vi "MAT Search Matrix.vi"(7 "offset in (-1: current position)":i64=-1, 8 "Error In":errorcluster, 10 "matrix name":string, 11 "Ref Num":refnum<file>) -> (0 "error out":errorcluster, 3 "Dup Ref Num":refnum<file>)   [LabVIEW 2013]
doc: "Searches matrix offset in the MAT file. It will set the read pointer to start of the matrix header."
uses:
  <vilib>/Utility/error.llb/Error Cluster From Error Code.vi
  <vilib>/ErrorRing/Error Ring.xnode
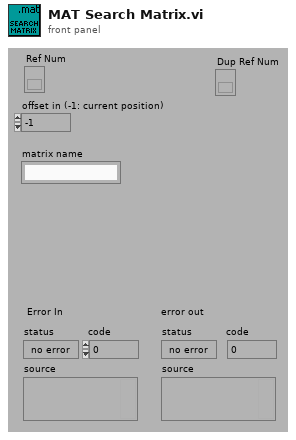
[diagram p1: front panel]
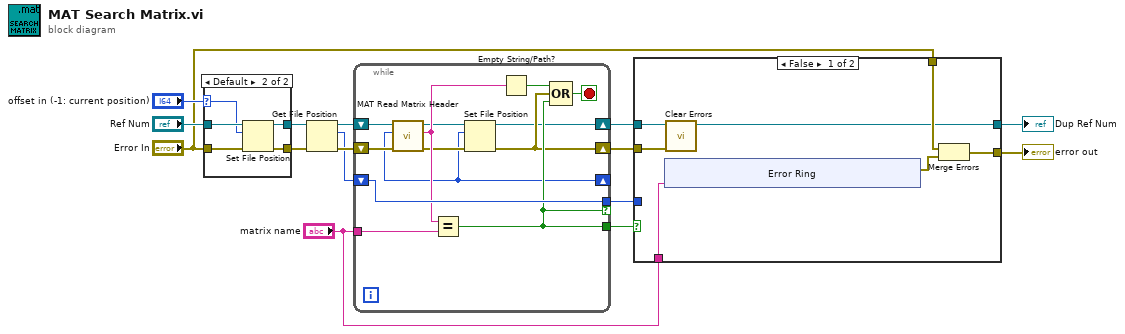
[diagram p0: block diagram]
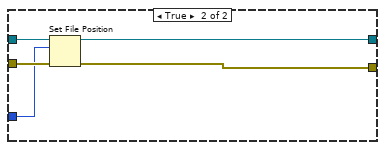
[diagram p2: hidden frame]
diagram:
  n1 = case shown="Default" "offset in (-1: current position)" {
    selector: "offset in (-1: current position)" -> [_ w18]
    tunnel: "Error In" -> [w16 w22]
    tunnel: [w16 w21] -> w13
    tunnel: [w17 w20] -> w12
    tunnel: "Ref Num" -> [w17 w19]
    frame -1 {
    }
    frame Default {
      n2 = Set File Position(offset (in bytes) (0)=w18, refnum=w19, error in=w22) -> (refnum out=w20:refnum<file>, error out=w21:errorcluster)  [unwired: 1 in]
    }
  }
  n3 = Get File Position(4:w13, 7:w12) -> (0:w11:errorcluster, 2:w9:i64, 3:w10:refnum<file>)
  n4 = while {
    shift-right: [w26] -> w7
    shift-left: w11 -> [w35]
    shift-right: [w24] -> w6
    shift-left: w10 -> [w34]
    shift-right: [w23] -> _
    shift-left: w9 -> [w32]
    tunnel: "matrix name" -> [w33]
    tunnel: [w32] -> w5 if=w28
    tunnel: [w28] -> w8
    stop <- w29 stop-if-true
    n5 = call "MAT Read Matrix Header.vi"("Error In"=w35, "Ref Num"=w34) -> ("error out"=w27:errorcluster, "Matrix Name"=w30:string, "Dup Ref Num"=w25:refnum<file>, "next variable offset"=w23:i64)  [unwired: 1 in, 5 out]
    n6 = Equal?(x=w30, y=w33) -> (x = y?=w28:bool)
    n7 = Set File Position(offset (in bytes) (0)=w23, refnum=w25, error in=w27) -> (refnum out=w24:refnum<file>, error out=w26:errorcluster)  [unwired: 1 in]
    n8 = Empty String/Path?(string/path=w30) -> (empty?=w31:bool)
    n9 = Compound Arithmetic op=OR(w31, w26, w28) -> (w29:bool)
  }
  n10 = case shown="False" w8 {
    tunnel: w7 -> [w37 w53]
    tunnel: w6 -> [w38 w52]
    tunnel: w5 -> [_ w51]
    tunnel: [w39 w50] -> w4
    tunnel: [w38 w49] -> w3
    tunnel: "Error In" -> [w40 _]
    tunnel: "matrix name" -> [w36 _]
    frame False {
      n11 = xnode "Error Ring"("parameter 0"=w36) -> ("error out"=w41:errorcluster)
      n12 = call <vilib>:"Clear Errors.vi"("error in (no error)"=w37) -> ()  [unwired: 6 in, 1 out]
      n13 = Merge Errors(w40, w41) -> (w39:errorcluster)
    }
    frame True {
      n14 = Set File Position(offset (in bytes) (0)=w51, refnum=w52, error in=w53) -> (refnum out=w49:refnum<file>, error out=w50:errorcluster)  [unwired: 1 in]
    }
  }
  "error out" <- w4
  "Dup Ref Num" <- w3
